vi "setConnected.vi"(8 "error in (no error)":errorcluster, 10 "connected":bool, 11 "Connection in":refnum<class "Connection.lvclass">) -> (0 "error out":errorcluster, 3 "Connection out":refnum<class "Connection.lvclass">)   [LabVIEW 2013, in "MQTT_Connection.lvlib" / "Connection.lvclass"]
uses:
  Connection.lvclass
  Connection.lvclass/Connection.ctl
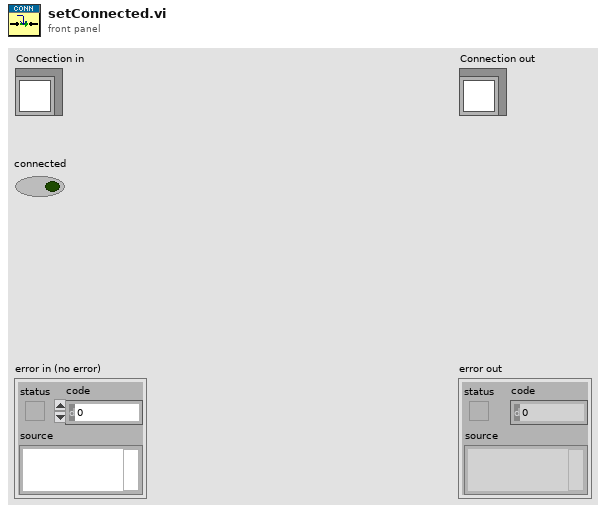
[diagram p1: front panel]
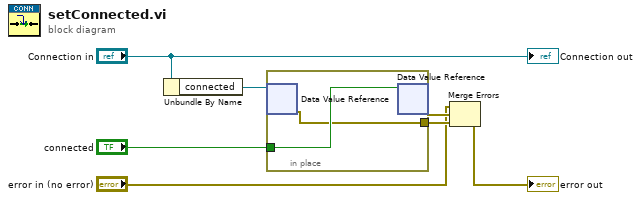
[diagram p0: block diagram]
diagram:
  n1 = Unbundle By Name("Connection in") -> ("connected"=w6:refnum<data-value>)
  n2 = in-place {
    in-place-border: "connected" -> [w9]
    in-place-border: [w8] -> w3
    n3 = in-place-dvr #1(w6) -> (w8:errorcluster)  [unwired: 1 out]
    n4 = in-place-dvr #1(w9) -> (w4:errorcluster)  [unwired: 1 out]
  }
  n5 = Merge Errors("error in (no error)", w4, w3) -> (→"error out":errorcluster)
  "Connection out" <- "Connection in"
